vi "LF_Initialise_And_GetParams.vi"() -> ()   [LabVIEW 2019]
uses:
  lightfield-automation-labview/LightField Automation.lvclass
panel:
  in  "Numeric":dbl
  out "size PL":i32
  out "size WL":i32
  out "XY Graph":cluster{"ColumnCalibration":dbl[], dbl[]}(graph)
  in  "Stop":bool
  out "DeltaE":dbl
  out "Image":dbl[][][](array[numeric])
  out "Intensity Graph":dbl[][](graph)
  out "Data":T1(array[cluster])
  in  "Frames":i32
  out "size(s)":i32
  out "ColumnCalibration":dbl[](array[numeric])
  out "Center Wavelength":dbl
  out "Current Grating":string
  out "Gratings":string[](array[string])
  out "Temperature (°C)":dbl
  out "Exposure Time (s)":dbl
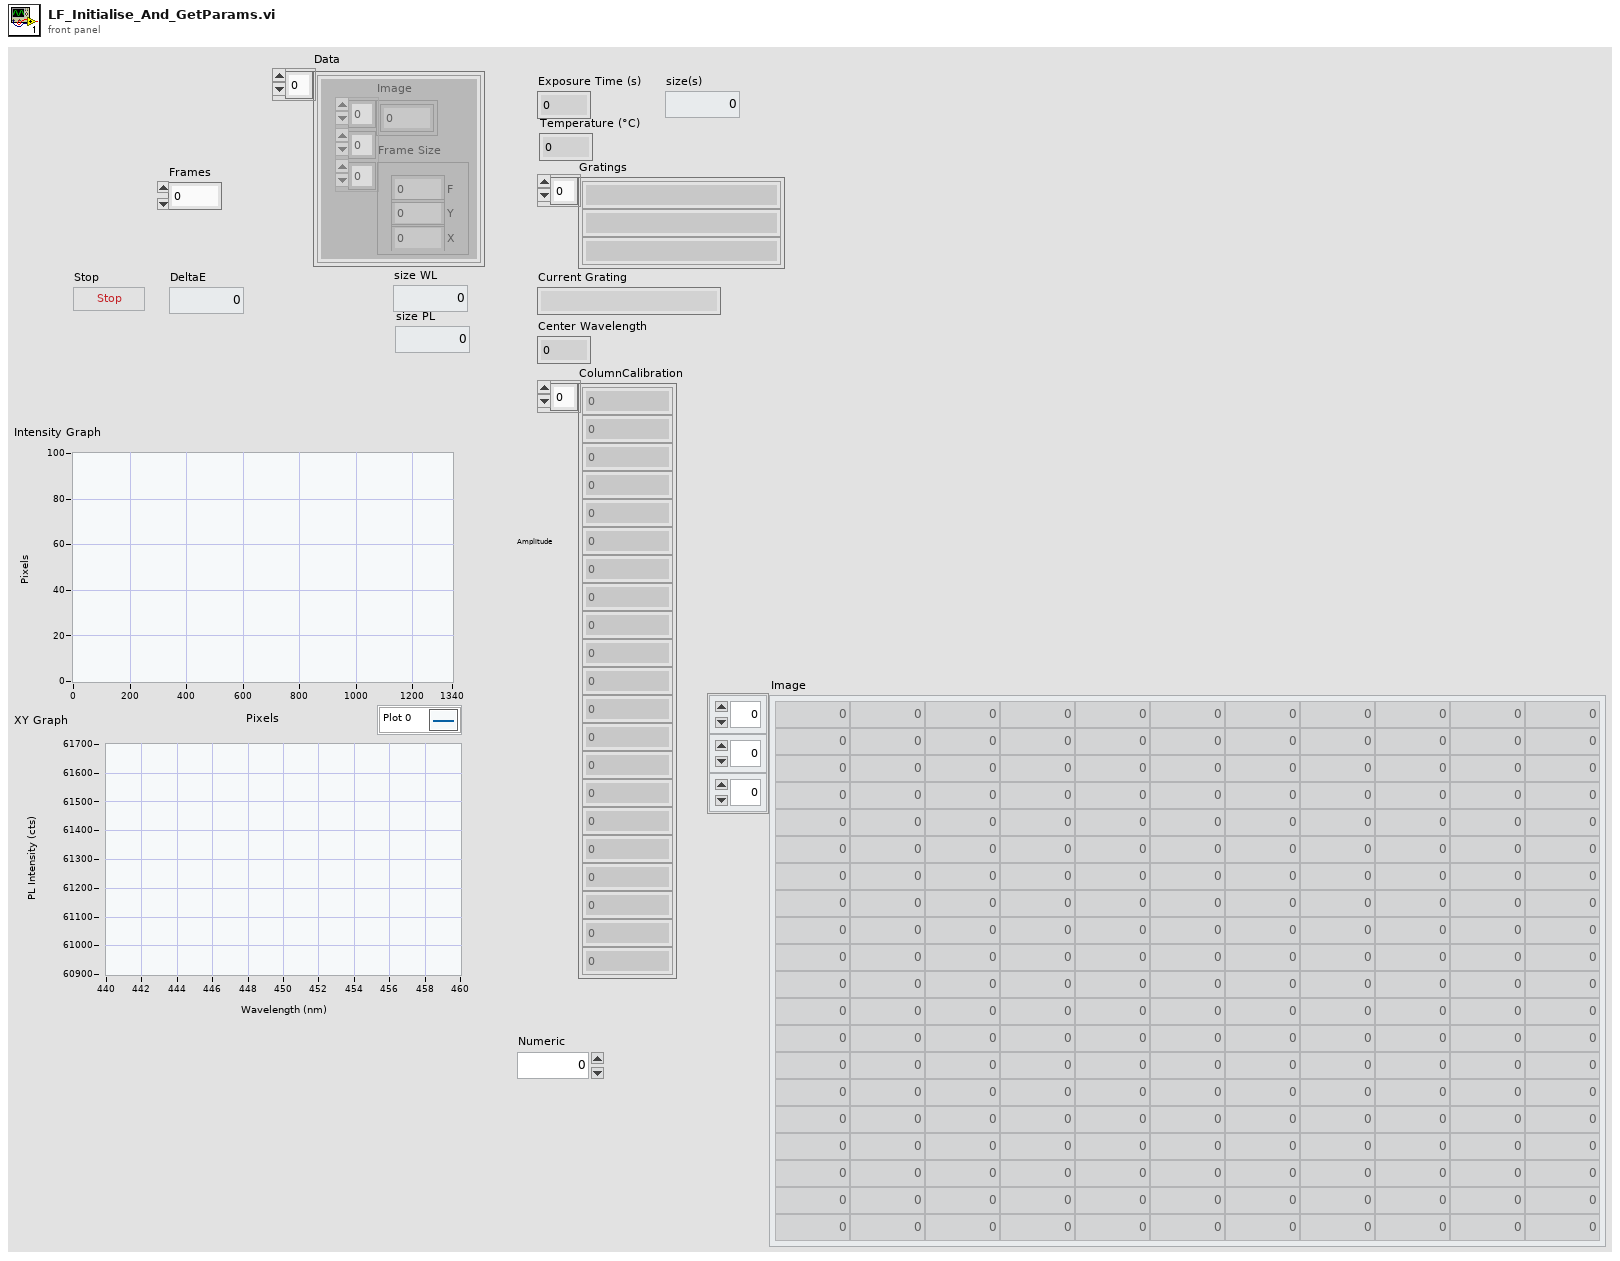
[diagram p1: front panel]
types:
  T1 = cluster{"Image":dbl[][][], "Frame Size":cluster{"F":i32, "Y":i32, "X":i32}}[]
  T2 = cluster{"Image":dbl[][][], "Frame Size":cluster{"F":i32, "Y":i32, "X":i32}}
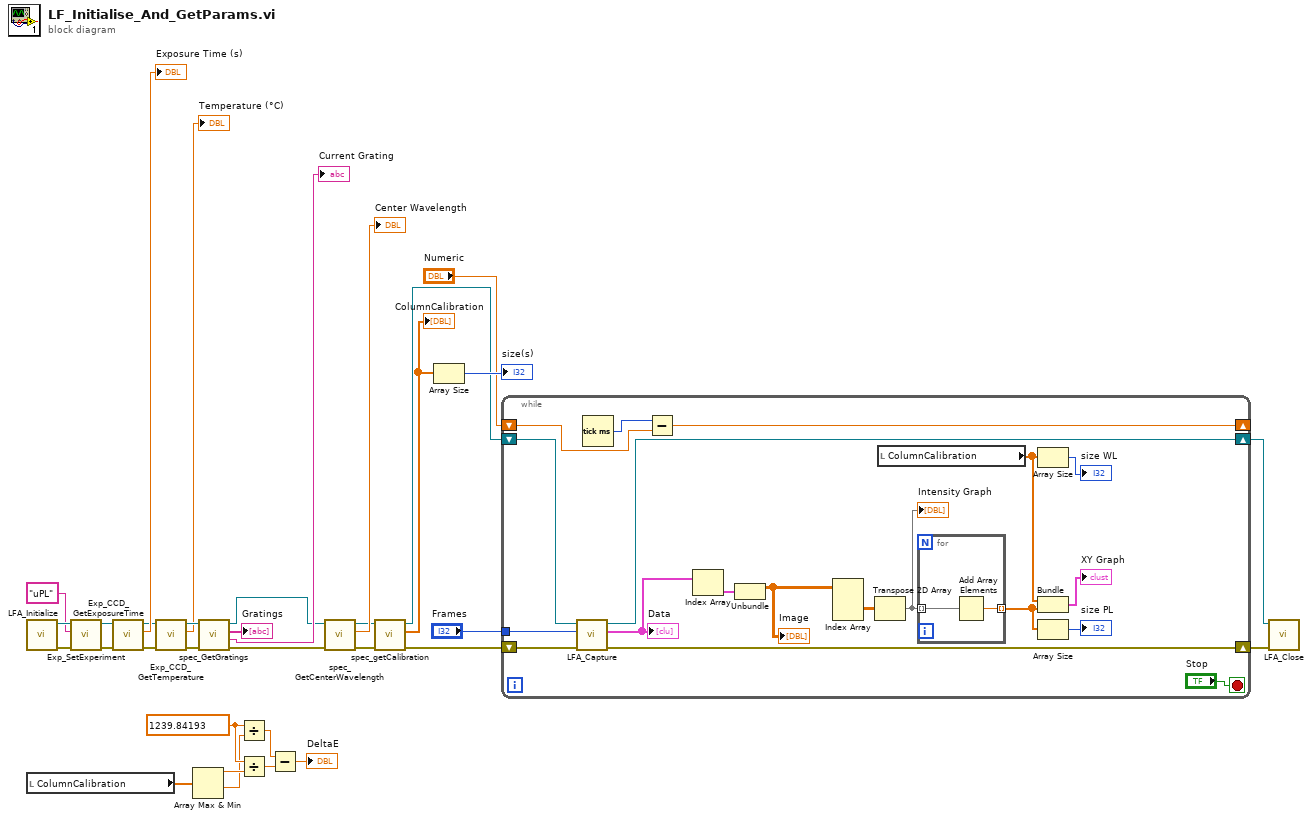
[diagram p0: block diagram]
diagram:
  w7 = 1239.84193
  n1 = call "LFA_Initialize.vi"() -> ("error out"=w32:errorcluster, "LightField Automation out"=w33:refnum<class "LightField Automation.lvclass">)  [unwired: 10 in]
  n2 = local read "ColumnCalibration"() -> (w8:dbl[])
  n3 = call "Exp_SetExperiment.vi"("error in (no error)"=w32, "ExperimentName"="uPL", "LightField Automation in"=w33) -> ("error out"=w29:errorcluster, "LightField Automation out"=w30:refnum<class "LightField Automation.lvclass">)  [unwired: 7 in]
  n4 = call "Exp_CCD_GetExposureTime.vi"("error in (no error)"=w29, "LightField Automation in"=w30) -> ("error out"=w24:errorcluster, "Exposure Time (s)"=→"Exposure Time (s)":dbl, "LightField Automation out"=w25:refnum<class "LightField Automation.lvclass">)  [unwired: 7 in]
  n5 = call "Exp_CCD_GetTemperature.vi"("error in (no error)"=w24, "LightField Automation in"=w25) -> ("error out"=w22:errorcluster, "Temperature (°C)"=→"Temperature (°C)":dbl, "LightField Automation out"=w23:refnum<class "LightField Automation.lvclass">)  [unwired: 7 in]
  n6 = Array Max & Min(array=w8) -> (max value=w6:dbl, min value=w5:dbl)  [unwired: 2 out]
  n7 = call "spec_GetGratings.vi"("error in (no error)"=w22, "LightField Automation in"=w23) -> ("error out"=w17:errorcluster, "Current Grating"=→"Current Grating":string, "Gratings"=→"Gratings":string[], "LightField Automation out"=w18:refnum<class "LightField Automation.lvclass">)  [unwired: 6 in]
  n8 = Divide(x=w7, y=w5) -> (x/y=w4:dbl)
  n9 = Divide(x=w7, y=w6) -> (x/y=w3:dbl)
  n10 = Subtract(x=w4, y=w3) -> (x-y=→"DeltaE":dbl)
  n11 = call "spec_GetCenterWavelength.vi"("error in (no error)"=w17, "LightField Automation in"=w18) -> ("error out"=w14:errorcluster, "Center Wavelenght"=→"Center Wavelength":dbl, "LightField Automation out"=w15:refnum<class "LightField Automation.lvclass">)  [unwired: 7 in]
  n12 = call "spec_getCalibration.vi"("error in (no error)"=w14, "LightField Automation in"=w15) -> ("error out"=w9:errorcluster, "ColumnCalibration"=w13:dbl[], "LightField Automation out"=w10:refnum<class "LightField Automation.lvclass">)  [unwired: 7 in]
  "ColumnCalibration" <- w13
  n13 = Array Size(array=w13) -> (size(s)=→"size(s)":i32)
  n14 = while {
    tunnel: "Frames" -> [w50]
    shift-right: [w52] -> w28
    shift-left: w10 -> [w49]
    shift-right: [w51] -> w27
    shift-left: w9 -> [w48]
    shift-right: [w34] -> _
    shift-left: "Numeric" -> [w35]
    stop <- "Stop" stop-if-true
    n15 = call "LFA_Capture.vi"("error in (no error)"=w48, "Frames"=w50, "LightField Automation in"=w49) -> ("error out"=w51:errorcluster, "Data"=w47:T1, "LightField Automation out"=w52:refnum<class "LightField Automation.lvclass">)  [unwired: 6 in]
    "Data" <- w47
    n16 = Tick Count (ms)() -> (millisecond timer value=w36:u32)
    n17 = Subtract(x=w36, y=w35) -> (x-y=w34:dbl)
    n18 = Index Array(array=w47) -> (element=w46:T2)  [unwired: 1 in]
    n19 = Unbundle(w46) -> ("Image"=w45:dbl[][][])  [unwired: 1 out]
    "Image" <- w45
    n20 = Index Array(array=w45) -> (element=w43:dbl[][])  [unwired: 3 in]
    n21 = Transpose 2D Array(2D array=w43) -> (transposed array=w41:dbl[][])
    "Intensity Graph" <- w41
    n22 = local read "ColumnCalibration"() -> (w40:dbl[])
    n23 = for {
      tunnel: w41 -> [w54] mode=indexing
      tunnel: [w53] -> w38 mode=indexing
      n24 = Add Array Elements(numeric array=w54) -> (sum=w53:dbl)
    }
    n25 = Array Size(array=w40) -> (size(s)=→"size WL":i32)
    n26 = Bundle("ColumnCalibration"=w40, w38) -> (→"XY Graph":cluster{"ColumnCalibration":dbl[], dbl[]})  [unwired: 1 in]
    n27 = Array Size(array=w38) -> (size(s)=→"size PL":i32)
  }
  n28 = call "LFA_Close.vi"("error in (no error)"=w27, "LightField Automation in"=w28) -> ()  [unwired: 8 in, 2 out]
